vi "Get Last Update String.vi"(8 "error in (no error)":errorcluster, 11 "WebProjectPanel in":refnum<class "WebProjectPanel.lvclass">) -> (0 "error out":errorcluster, 2 "Last Update":string, 3 "WebProjectPanel out":refnum<class "WebProjectPanel.lvclass">)   [LabVIEW 2020, in "PicoG-Processor.lvlib" / "WebProjectPanel.lvclass"]
uses:
  WebProjectPanel.lvclass
  WebProjectPanel.lvclass/WebProjectPanel.ctl
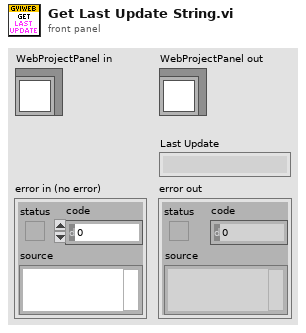
[diagram p1: front panel]
types:
  T1 = typedef "PicoG-Processor.lvlib/WebProjectPanel.lvclass/Ref Data.ctl" = cluster{"Last Update":dbl, "Path":path, "App Name":string, "Build Present":bool, "Deploy":refnum<user-event>}
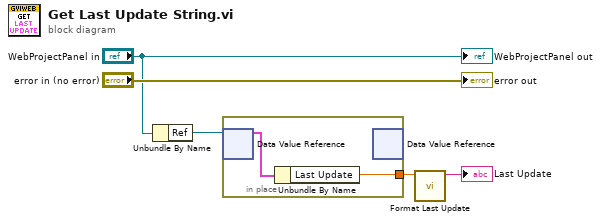
[diagram p0: block diagram]
diagram:
  n1 = Unbundle By Name("WebProjectPanel in") -> ("Ref"=w4:refnum<data-value>)
  n2 = in-place {
    in-place-border: [w6] -> w2
    n3 = in-place-dvr #1(w4) -> (w7:T1)  [unwired: 1 out]
    n4 = Unbundle By Name(w7) -> ("Last Update"=w6:dbl)
    n5 = in-place-dvr #1() -> ()  [unwired: 1 in, 2 out]
  }
  n6 = call "Format Last Update.vi"("Last Update"=w2) -> ("Last Update String"=→"Last Update":string)  [unwired: 10 in]
  "error out" <- "error in (no error)"
  "WebProjectPanel out" <- "WebProjectPanel in"
